vi "Arduino input-output.vi"(0 "VISA resource name":refnum<visa-resource-name>="COM18", 1 "Sets to read":u32=1, 2 "Error in":errorcluster) -> (3 "VISA resource out":refnum<visa-resource-name>="COM18", 4 "Channel names":string[](array[string]), 5 "Output":dbl[][](array[numeric]), 6 "Error out":errorcluster)   [LabVIEW 2014]
panel:
  out "String":string
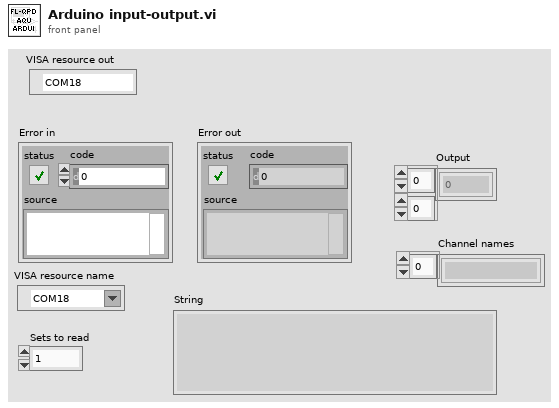
[diagram p1: front panel]
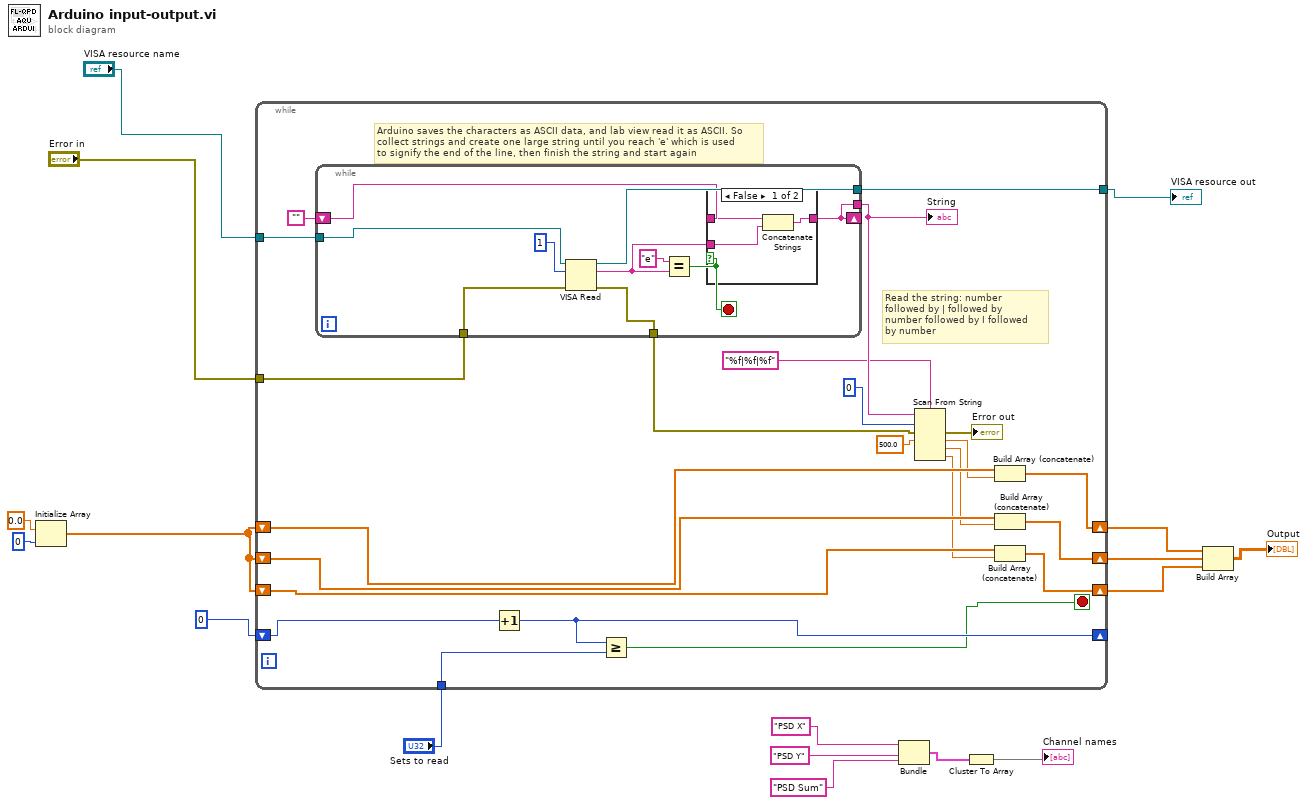
[diagram p0: block diagram]
diagram:
  n1 = Initialize Array(0.0, 0) -> (w13:dbl[])
  n2 = while {
    tunnel: "VISA resource name" -> [w32]
    tunnel: [w40] -> w1
    tunnel: "Error in" -> [w33]
    shift-right: [w30] -> _
    shift-left: u32 0 -> [w31]
    tunnel: "Sets to read" -> [w29]
    shift-right: [w22] -> w10
    shift-left: w13 -> [w28]
    shift-right: [w21] -> w9
    shift-left: w13 -> [w26]
    shift-right: [w20] -> w8
    shift-left: w13 -> [w24]
    stop <- w18 stop-if-true
    # "Read the string: number \nfollowed by | followed by\nnumber followed by I followed \nby number"
    # "Arduino saves the characters as ASCII data, and lab view read it as ASCII. So\ncollect strings and create one large string until you reach 'e' which is used \nto signify the end of the line, then finish the string and start again"
    n3 = while {
      tunnel: [w43] -> w38
      tunnel: w32 -> [w50]
      tunnel: [w48] -> w40
      shift-right: [w43] -> _
      shift-left: "" -> [w44]
      tunnel: w33 -> [w42]
      tunnel: [w41] -> w19
      stop <- w45 stop-if-true
      n4 = VISA Read(VISA resource name=w50, byte count=1, error in (no error)=w42) -> (VISA resource name out=w48:refnum<visa-resource-name>, read buffer=w46:string, error out=w41:errorcluster)  [unwired: 1 out]
      n5 = Equal?(x="e", y=w46) -> (x = y?=w45:bool)
      n6 = case shown="False" w45 {
        tunnel: w44 -> [w53 w54]
        tunnel: w46 -> [w52 _]
        tunnel: [w51 w54] -> w43
        frame False {
          n7 = Concatenate Strings(w53, w52) -> (w51:string)
        }
        frame True {
        }
      }
    }
    "String" <- w38
    n8 = Increment(x=w31) -> (x+1=w30:u32)
    n9 = Greater Or Equal?(x=w30, y=w29) -> (x >= y?=w18:bool)
    n10 = Scan From String(format string="%f|%f|%f", input string=w38, initial scan location=0, error in=w19, default 1=500.0) -> (error out=→"Error out":errorcluster, output 1=w27:dbl, output 2=w25:dbl, output 3=w23:dbl)  [unwired: 2 in, 2 out]
    n11 = Build Array (concatenate)(w28, w27) -> (w22:dbl[])
    n12 = Build Array (concatenate)(w26, w25) -> (w21:dbl[])
    n13 = Build Array (concatenate)(w24, w23) -> (w20:dbl[])
  }
  "VISA resource out" <- w1
  n14 = Bundle("PSD X", "PSD Y", "PSD Sum") -> (w3:cluster{string, string, string})  [unwired: 1 out]
  n15 = Cluster To Array(cluster=w3) -> (array=→"Channel names":string[])
  n16 = Build Array(w10, w9, w8) -> (→"Output":dbl[][])
